vi "H-cube - MAIN.vi"() -> ()   [LabVIEW 2019]
doc: "Use this template to build a producer/consumer design pattern with events to produce queue items. Use this design pattern instead of the User Interface Event Handler pattern for user interfaces when you want to execute code asynchronously in response to an event without slowing the user interface responsiveness."
uses:
  MAIN STATUS.ctl
  FPGA/FPGA.ctl
  FPGA/ResultSweep.vi
  <vilib>/Utility/file.llb/Write Delimited Spreadsheet (DBL).vi
  FPGA/FPGA.lvlib
panel:
  in  "ClearFIFO":bool
  in  "FIFO EN":bool
  out "FIFO":string[][](array[string])
  in  "Add FIFO":bool
  in  "Continuous save":bool
  in  "File name":string
  in  "Path":path
  in  "Incremental Save":bool
  in  "Continuous run":bool
  in  "raw data slice":bool
  in  "Settling at step time":enum16{"99%", "99,9%"}(ring)=enum."99,9%"
  in  "Lockin filter order":u32=2 min=1 max=4
  out "Averaging":bool
  in  "Averaging":bool
  out "Averaging prefered":bool
  in  "Auto MA selection":bool
  out "Number of steps":i32=1
  in  "Save":bool caption="OK Button"
  in  "Digital Gain":i32(ring) items=["1", "2", "4", "8", "16", "32", "64"]
  out "XY Graph 2":cluster{dbl[], dbl[]}(graph)
  out "XY Graph":cluster{dbl[], dbl[]}(graph)
  in  "DAC-ADC Latency":u16=80 min=1 max=1024 step=1
  out "Acquiring":bool
  in  "Lock-in":bool=TRUE
  in  "Amplitude [mVpp]":dbl=100.0 min=0.0 max=5000.0
  in  "connect":bool
  out "Connected":bool=TRUE
  out "Sweep speed [Hz/s]":dbl=999.9995081132196
  out "Time for step [ms]":dbl=100.0
  in  "Discrete\nsweep":bool=TRUE
  in  "Freq. step [Hz]":dbl=100.0 min=0.0
  in  "Sweep duration [s]":dbl=10.0 min=0.0
  in  "Stop freq. [Hz]":dbl=20000.0
  in  "Start freq. [Hz]":dbl=10000.0
  in  "exit":bool
  in  "stop":bool
  in  "start":bool
  # "SWEEP\nCONTROLS"
  # "ADVANCED\nCONTROLS"
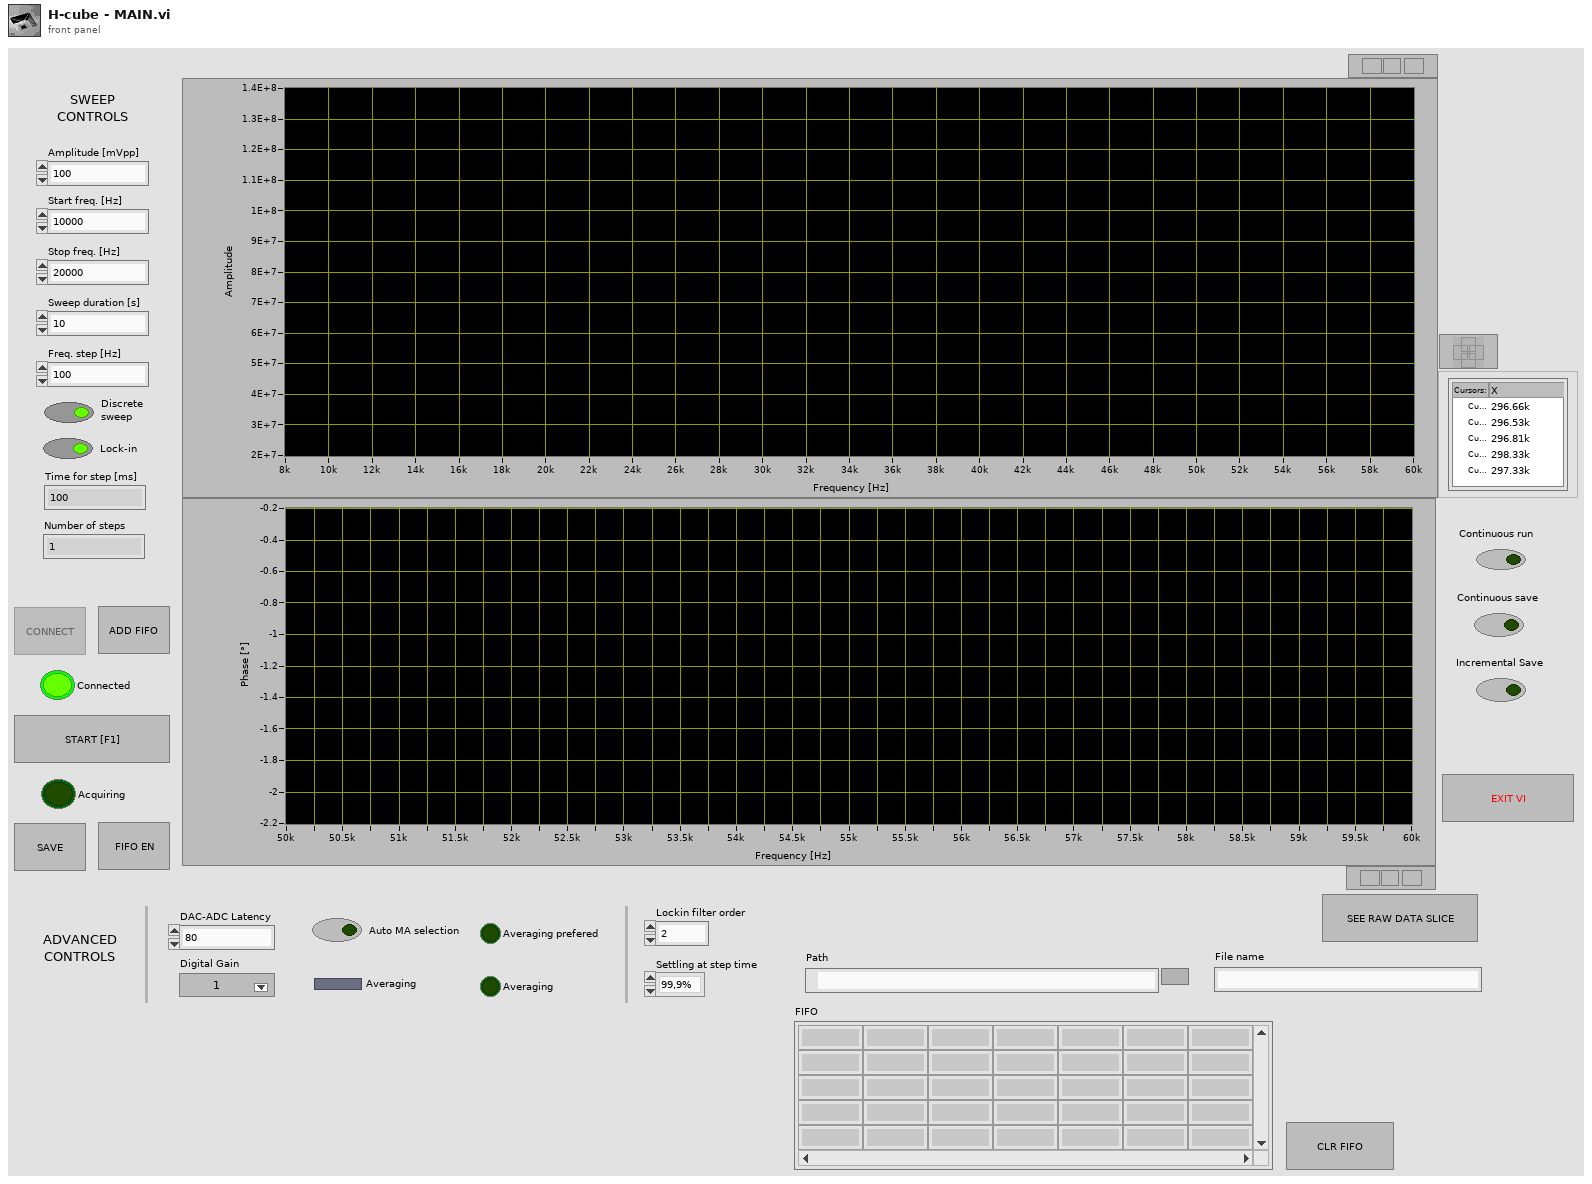
[diagram p1: front panel]
types:
  T1 = enum8{"Enabled", "Disabled", "Disabled and Grayed Out"}
  T2 = typedef "MAIN STATUS.ctl" = enum16{"IDLE", "Refresh UI", "ChangeParameters", "StopSweep", "StartSweep", "RawData", "CheckParameters", "SendParameters", "Connect", "AddFIFO", "Save", "Quit", "ClrFIFO", "StartSweepFIFO"}
  T3 = typedef "FPGA.lvlib/FPGA.ctl" = cluster{"Start freq. [Hz]":dbl, "Sweep duration [s]":dbl, "Freq. step [Hz]":dbl, "DAC Sample Rate":dbl, "ADC Sample Rate":dbl, "CMD port":u16, "DFAST port":u16, "CMD ID":refnum<k16>, "DFAST ID":refnum<k16>, "CMD error out":errorcluster, "FPGA IP":string, "DFAST error out ":errorcluster, "Stop freq. [Hz]":dbl, "Discrete sweep":bool, "Initial NCO":u32, "Difference NCO":i32, "step NCO":i64, "Final NCO":u32, "clocks for step":u32, "demodulation":bool, "NCO Phase Precision":u32, "NCO Sample Rate":dbl, "Time for step [s]":dbl, "NCO freq. resolution":dbl, "Sweep speed [Hz/s]":dbl, "Connected":bool, "Slew Rate [V/us]":dbl, "Parameters_ok":bool, "Amplitude [mVpp]":dbl, "Scale Factor":fxp<+,16,0>, "Acquiring":bool, "DAC-ADC Latency":u16, "Digital Gain":i32, "Number of steps":i32, "Averaging preferred":bool, "Filter Order":u32, "Settling":enum16{"99%", "99,9%"}, "FIFO":cluster{"Start freq. [Hz]":dbl, "Sweep duration [s]":dbl, "Freq. step [Hz]":dbl, "Stop freq. [Hz]":dbl, "Time for step [s]":dbl, "Amplitude [mVpp]":dbl, "Number of steps":i32}[]}
  T4 = cluster{"CMD port":u16, "CMD ID":refnum<k16>, "DFAST port":u16, "DFAST ID":refnum<k16>, "CMD error out":errorcluster, "DFAST error out ":errorcluster, "FPGA IP":string}
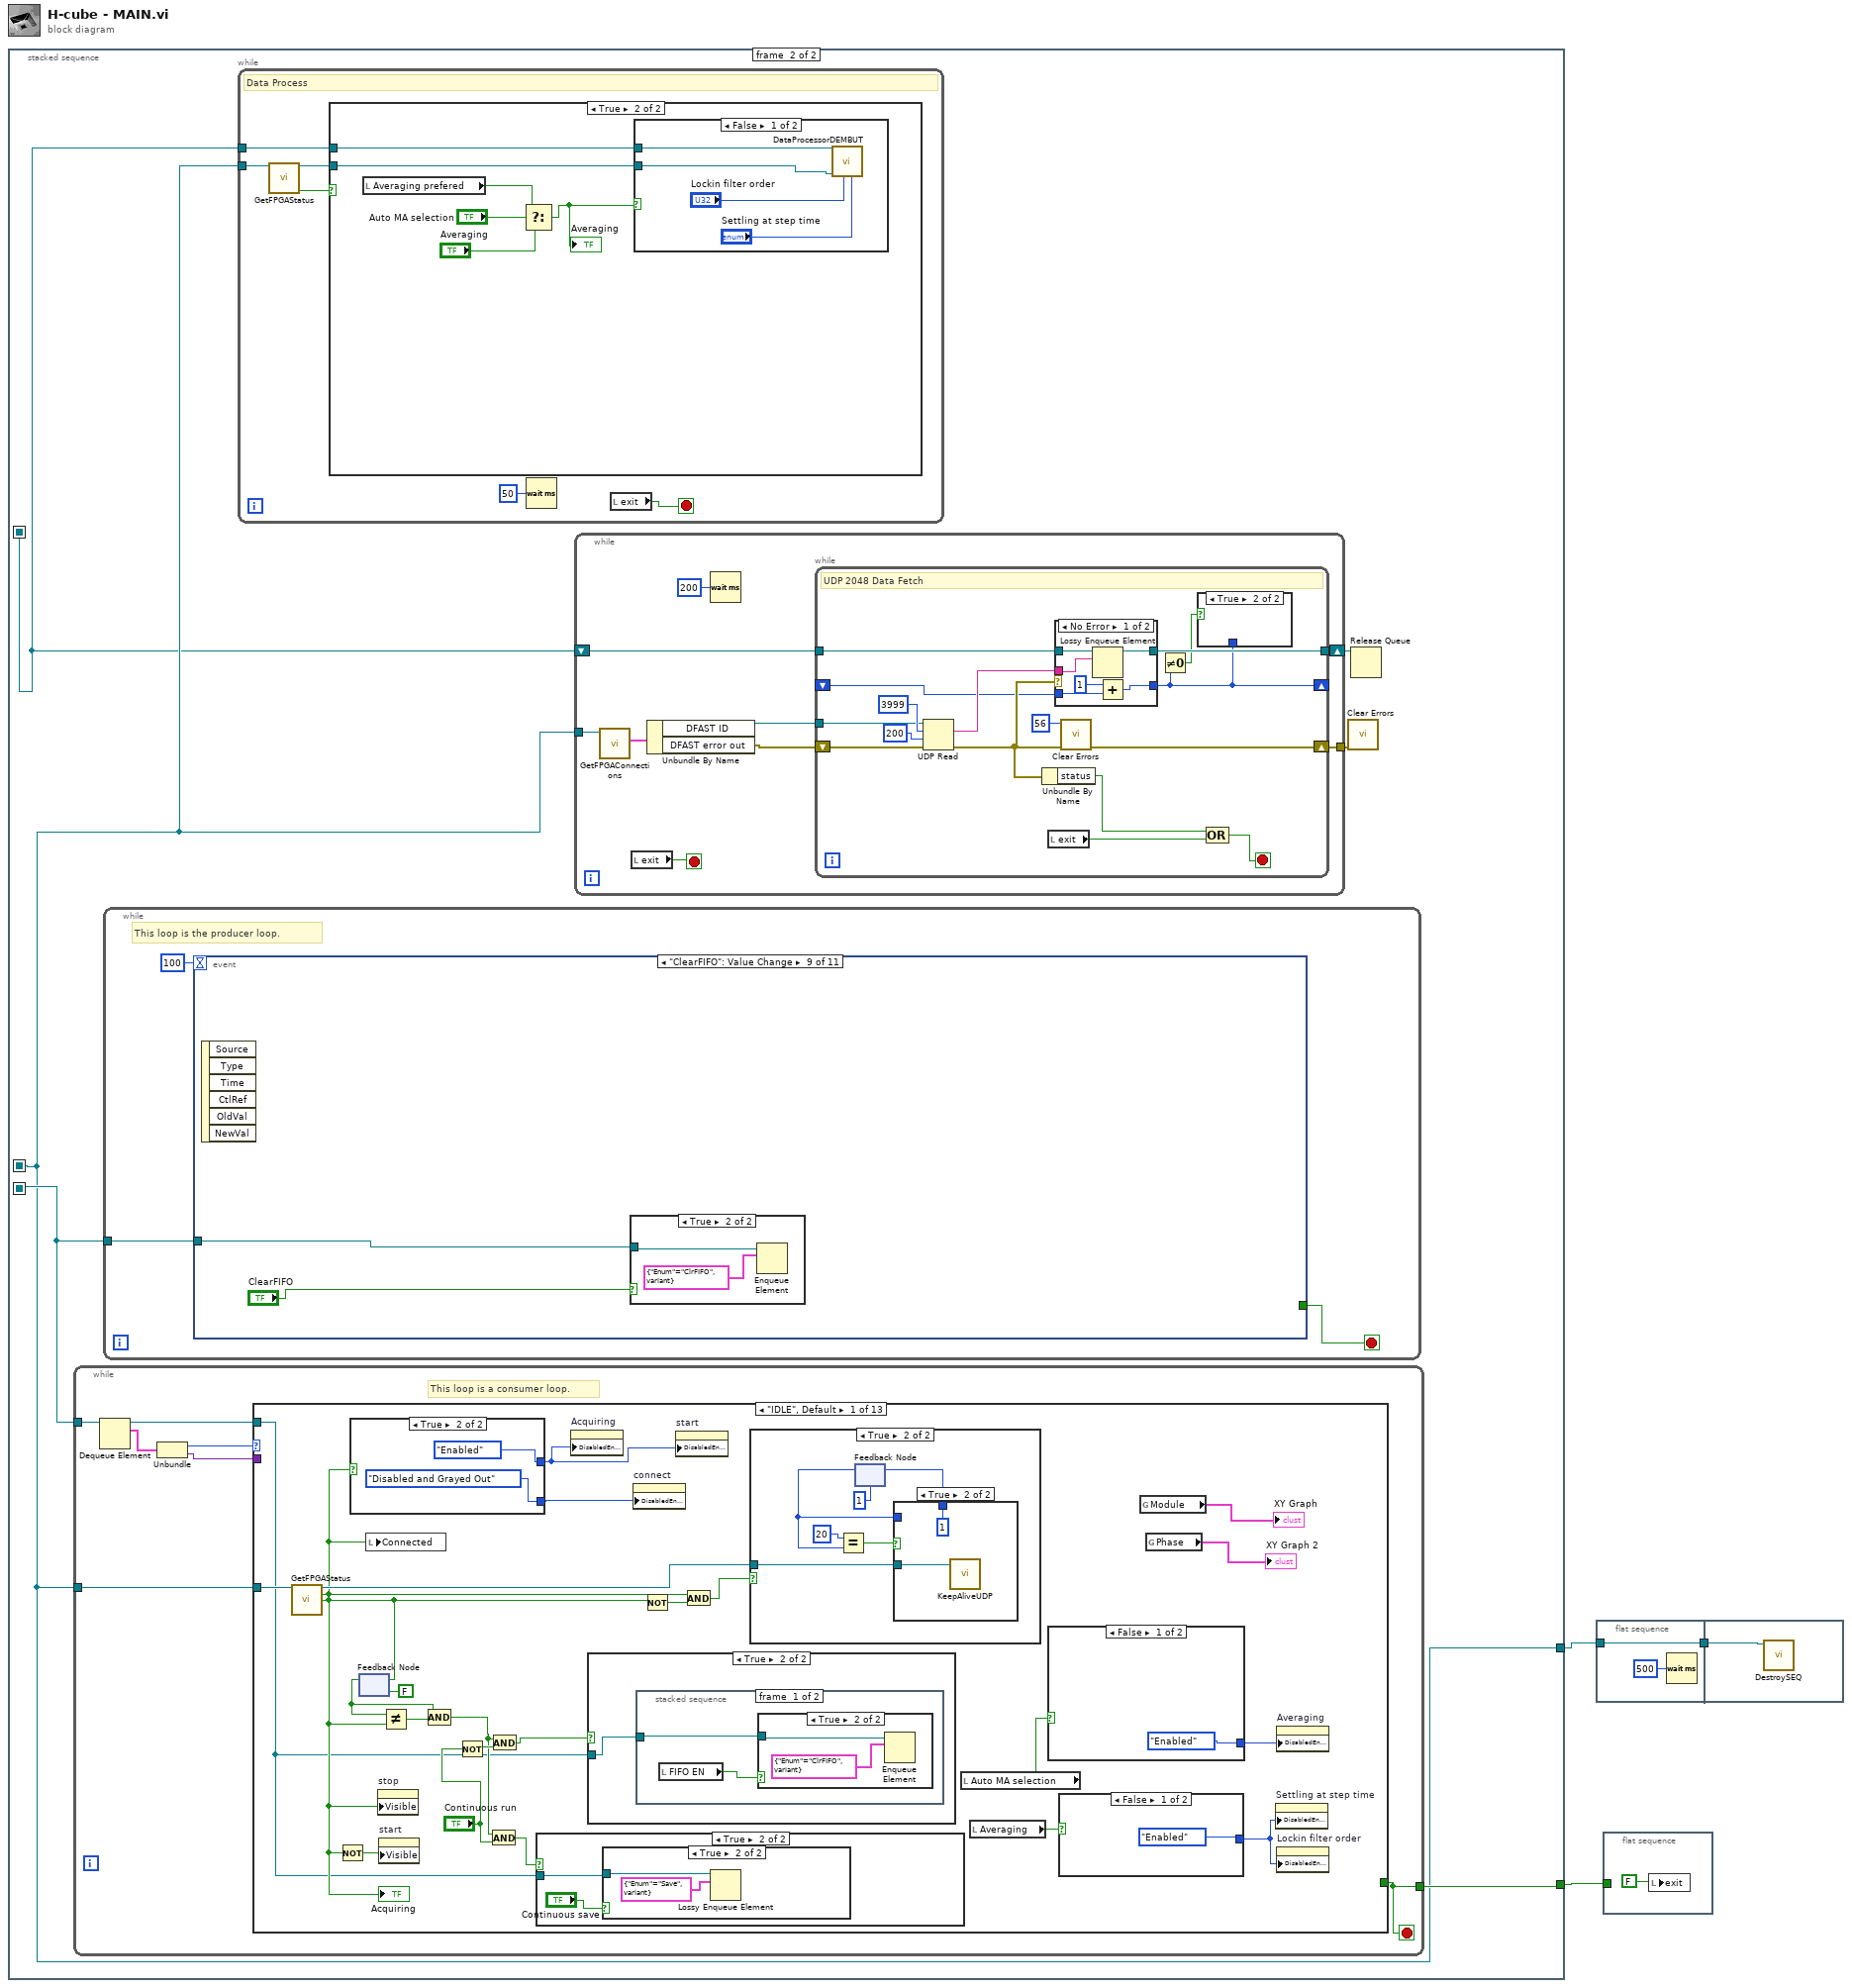
[diagram p0: block diagram]
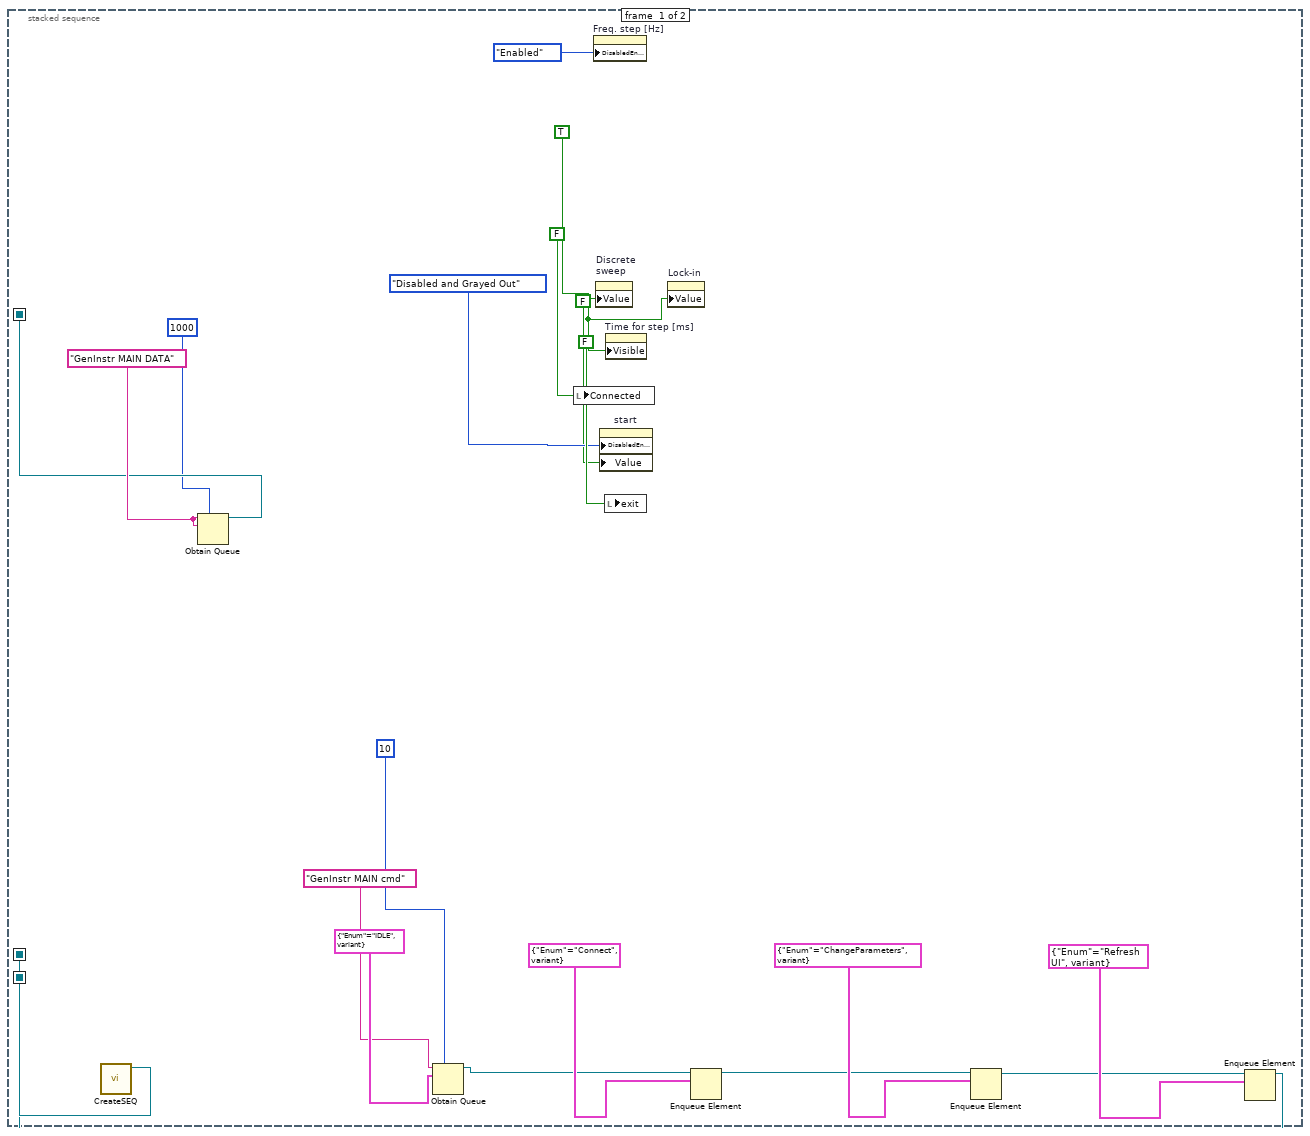
[diagram p2: hidden frame]
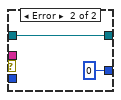
[diagram p4: hidden frame]
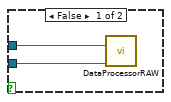
[diagram p5: hidden frame]
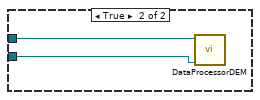
[diagram p6: hidden frame]
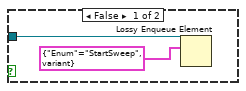
[diagram p8: hidden frame]
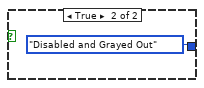
[diagram p9: hidden frame]
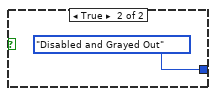
[diagram p10: hidden frame]
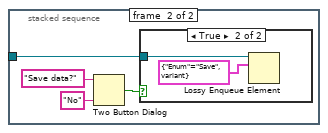
[diagram p13: hidden frame]
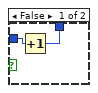
[diagram p16: hidden frame]
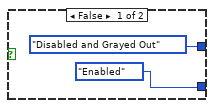
[diagram p17: hidden frame]
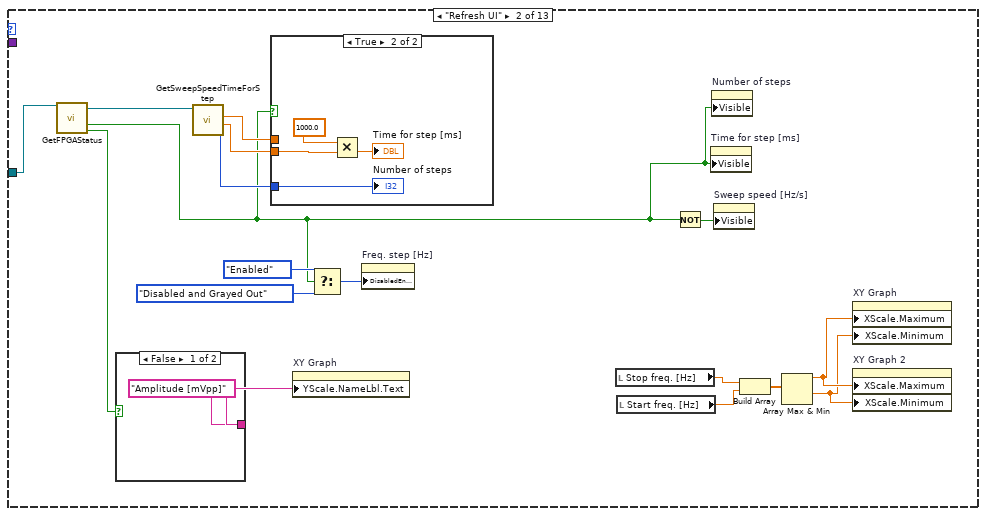
[diagram p18: hidden frame]
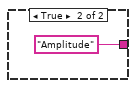
[diagram p19: hidden frame]
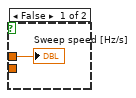
[diagram p20: hidden frame]
diagram:
  n1 = stacked-sequence {
    seq-local: [w11 _] -> [_ w29]
    seq-local: [w19 _] -> [_ w24]
    seq-local: [w15 _] -> [_ w25]
    tunnel: [_ w28] -> w3
    tunnel: [_ w25] -> w2
    frame #0 {
      w4 = TRUE ("Discrete\nsweep")
      w20 = "GenInstr MAIN DATA" ("name (unnamed)")
      n2 = call "CreateSEQ.vi"() -> ("FPGA out"=w15:refnum<queue>)  [unwired: 10 in, 1 out]
      n3 = Obtain Queue(max queue size (-1, unlimited)=1000, name (unnamed)=w20, element data type=w20) -> (queue out=w19:refnum<queue>)  [unwired: 2 in, 2 out]
      n4 = Obtain Queue(max queue size (-1, unlimited)=10, name (unnamed)="GenInstr MAIN cmd", element data type=cluster{"Enum":T2, variant} {"Enum"=enum."IDLE", variant}) -> (queue out=w9:refnum<queue>)  [unwired: 2 in, 2 out]
      n5 = local write "Connected"(FALSE ("Connected")) -> ()
      n6 = property on="Freq. step [Hz]" class="DigNum (strict)"("DisabledEnum"=T1."Enabled" ("Disabled")) -> ()  [unwired: 2 in, 2 out]
      n7 = property on="Discrete\nsweep" class="Bool (strict)"("Value"=w4) -> ()  [unwired: 2 in, 2 out]
      n8 = property on="start" class="Bool"("DisabledEnum"=T1."Disabled and Grayed Out" ("Disabled"), "Value"=FALSE ("start")) -> ()  [unwired: 2 in, 2 out]
      n9 = local write "exit"(FALSE ("stop")) -> ()
      n10 = property on="Time for step [ms]" class="DigNum (strict)"("Visible"=w4) -> ()  [unwired: 2 in, 2 out]
      n11 = property on="Lock-in" class="Bool (strict)"("Value"=w4) -> ()  [unwired: 2 in, 2 out]
      n12 = Enqueue Element(queue=w9, element=cluster{"Enum":T2, variant} {"Enum"=enum."Connect", variant}) -> (queue out=w8:refnum<queue>)  [unwired: 2 in, 2 out]
      n13 = Enqueue Element(queue=w8, element=cluster{"Enum":T2, variant} {"Enum"=enum."ChangeParameters", variant}) -> (queue out=w12:refnum<queue>)  [unwired: 2 in, 2 out]
      n14 = Enqueue Element(queue=w12, element=cluster{"Enum":T2, variant} {"Enum"=enum."Refresh UI", variant}) -> (queue out=w11:refnum<queue>)  [unwired: 2 in, 2 out]
    }
    frame #1 {
      n15 = while {
        tunnel: w29 -> [w84]
        tunnel: [w86] -> w28
        tunnel: w25 -> [w85]
        stop <- w86 stop-if-true
        # "This loop is a consumer loop."
        n16 = Dequeue Element(queue=w84) -> (queue out=w83:refnum<queue>, element=w89:cluster{"Enum":T2, variant})  [unwired: 2 in, 2 out]
        n17 = Unbundle(w89) -> ("Enum"=w88:T2, w87:variant)
        n18 = case shown="\"IDLE\", Default" w88 {
          tunnel: [_ _ TRUE _ _ _ _ _ _ _ _ _ _] -> w86
          tunnel: w87 -> [_ _ _ _ _ _ _ _ _ _ _ _ _]
          tunnel: w85 -> [w113 w158 w175 _ w219 w232 w239 _ w246 _ w253 w256 w258]
          tunnel: w83 -> [w90 _ _ w183 _ w230 _ _ _ _ _ _ _]
          frame "IDLE", Default {
            n19 = call "GetFPGAStatus.vi"("FPGA in"=w113) -> ("FPGA out"=w110:refnum<queue>, "Connected"=w97:bool, "Acquiring"=w105:bool)  [unwired: 9 in, 3 out]
            "Acquiring" <- w105
            n20 = Not(x=w105) -> (.not. x?=w107:bool)
            n21 = case shown="True" w97 {
              tunnel: [T1."Disabled and Grayed Out" ("Disabled") T1."Enabled" ("Disabled")] -> w98
              tunnel: [T1."Enabled" ("Disabled") T1."Disabled and Grayed Out" ("Disabled")] -> w96
              frame False {
              }
              frame True {
              }
            }
            n22 = feedback-in #1(w105) -> ()
            n23 = feedback #1(FALSE ("Acquiring")) -> (w104:bool)
            n24 = local write "Connected"(w97) -> ()
            n25 = property on="stop" class="Bool"("Visible"=w105) -> ()  [unwired: 2 in, 2 out]
            n26 = property on="start" class="Bool"("Visible"=w107) -> ()  [unwired: 2 in, 2 out]
            n27 = Not Equal?(x=w104, y=w105) -> (x != y?=w103:bool)
            n28 = Compound Arithmetic op=AND(w104, w103) -> (w92:bool)
            n29 = Not(x="Continuous run") -> (.not. x?=w94:bool)
            n30 = And(x=w92, y="Continuous run") -> (x .and. y?=w91:bool)
            n31 = And(x=w92, y=w94) -> (x .and. y?=w95:bool)
            n32 = case shown="True" w91 {
              tunnel: w90 -> [_ w114]
              frame False {
              }
              frame True {
                n33 = case shown="True" "Continuous save" {
                  tunnel: w114 -> [w116 w118]
                  frame False {
                    n34 = Lossy Enqueue Element(queue=w116, element=cluster{"Enum":T2, variant} {"Enum"=enum."StartSweep", variant}) -> ()  [unwired: 1 in, 4 out]
                  }
                  frame True {
                    n35 = Lossy Enqueue Element(queue=w118, element=cluster{"Enum":T2, variant} {"Enum"=enum."Save", variant}) -> ()  [unwired: 1 in, 4 out]
                  }
                }
              }
            }
            n36 = property on="Acquiring" class="Bool (strict)"("DisabledEnum"=w98) -> ()  [unwired: 2 in, 2 out]
            n37 = case shown="True" w95 {
              tunnel: w90 -> [_ w124]
              frame False {
              }
              frame True {
                n38 = stacked-sequence {
                  tunnel: w124 -> [w126 w129]
                  frame #0 {
                    n39 = local read "FIFO EN"() -> (w125:bool)
                    n40 = case shown="True" w125 {
                      tunnel: w126 -> [_ w127]
                      frame False {
                      }
                      frame True {
                        n41 = Enqueue Element(queue=w127, element=cluster{"Enum":T2, variant} {"Enum"=enum."ClrFIFO", variant}) -> ()  [unwired: 2 in, 3 out]
                      }
                    }
                  }
                  frame #1 {
                    n42 = Two Button Dialog(message="Save data?", 1:"No" ("F button name (\"Cancel\")")) -> (T button?=w130:bool)  [unwired: 1 in]
                    n43 = case shown="True" w130 {
                      tunnel: w129 -> [_ w133]
                      frame False {
                      }
                      frame True {
                        n44 = Lossy Enqueue Element(queue=w133, element=cluster{"Enum":T2, variant} {"Enum"=enum."Save", variant}) -> ()  [unwired: 1 in, 4 out]
                      }
                    }
                  }
                }
              }
            }
            n45 = property on="connect" class="Bool"("DisabledEnum"=w96) -> ()  [unwired: 2 in, 2 out]
            n46 = Not(x=w105) -> (.not. x?=w111:bool)
            n47 = property on="start" class="Bool"("DisabledEnum"=w98) -> ()  [unwired: 2 in, 2 out]
            n48 = And(x=w97, y=w111) -> (x .and. y?=w112:bool)
            n49 = case shown="True" w112 {
              tunnel: w110 -> [_ w136]
              frame False {
              }
              frame True {
                n50 = feedback #2(1 ("y")) -> (w135:i32)
                n51 = Equal?(x=20 ("y"), y=w135) -> (x = y?=w138:bool)
                n52 = case shown="True" w138 {
                  tunnel: [w141 1] -> w137
                  tunnel: w135 -> [w142 _]
                  tunnel: w136 -> [_ w144]
                  frame False {
                    n53 = Increment(x=w142) -> (x+1=w141:i32)
                  }
                  frame True {
                    n54 = call "KeepAliveUDP.vi"("FPGA in"=w144) -> ()  [unwired: 10 in, 1 out]
                  }
                }
                n55 = feedback-in #2(w137) -> ()
              }
            }
            n56 = local read "Auto MA selection"() -> (w100:bool)
            n57 = local read "Averaging"() -> (w102:bool)
            n58 = case shown="False" w100 {
              tunnel: [T1."Enabled" ("Disabled") T1."Disabled and Grayed Out" ("Disabled")] -> w101
              frame False {
              }
              frame True {
              }
            }
            n59 = case shown="False" w102 {
              tunnel: [T1."Enabled" ("Disabled") T1."Disabled and Grayed Out" ("Disabled")] -> w99
              frame False {
              }
              frame True {
              }
            }
            n60 = global read "ResultSweep.vi" "Module"() -> (→"XY Graph":cluster{dbl[], dbl[]})
            n61 = global read "ResultSweep.vi" "Phase"() -> (→"XY Graph 2":cluster{dbl[], dbl[]})
            n62 = property on="Settling at step time" class="Enum (strict)"("DisabledEnum"=w99) -> ()  [unwired: 2 in, 2 out]
            n63 = property on="Averaging" class="Bool (strict)"("DisabledEnum"=w101) -> ()  [unwired: 2 in, 2 out]
            n64 = property on="Lockin filter order" class="DigNum (strict)"("DisabledEnum"=w99) -> ()  [unwired: 2 in, 2 out]
          }
          frame "Refresh UI" {
            n65 = call "GetFPGAStatus.vi"("FPGA in"=w158) -> ("FPGA out"=w157:refnum<queue>, "Discrete Sweep"=w149:bool, "Demodulation"=w156:bool)  [unwired: 9 in, 3 out]
            n66 = case shown="False" w156 {
              tunnel: ["Amplitude [mVpp]" ("X Scale.Name Label.Text") "Amplitude" ("X Scale.Name Label.Text")] -> w159
              frame False {
              }
              frame True {
              }
            }
            n67 = call "GetSweepSpeedTimeForStep.vi"("FPGA in"=w157) -> ("Number of steps"=w150:i32, "Time for step [s]"=w162:dbl, "Sweep speed [Hz/s]"=w160:dbl)  [unwired: 7 in, 1 out]
            n68 = case shown="True" w149 {
              tunnel: w162 -> [_ w172]
              tunnel: w160 -> [w168 _]
              tunnel: w150 -> [_ w169]
              frame False {
                "Sweep speed [Hz/s]" <- w168
              }
              frame True {
                n69 = Multiply(x=1000.0, y=w172) -> (x*y=→"Time for step [ms]":dbl)
                "Number of steps" <- w169
              }
            }
            n70 = property on="XY Graph" class="XYGraph (strict)"("YScale.NameLbl.Text"=w159) -> ()  [unwired: 2 in, 2 out]
            n71 = Select(t=T1."Enabled", s=w149, f=T1."Disabled and Grayed Out" ("Disabled")) -> (s? t:f=w165:T1)
            n72 = property on="Freq. step [Hz]" class="DigNum (strict)"("DisabledEnum"=w165) -> ()  [unwired: 2 in, 2 out]
            n73 = local read "Stop freq. [Hz]"() -> (w154:dbl)
            n74 = local read "Start freq. [Hz]"() -> (w153:dbl)
            n75 = Not(x=w149) -> (.not. x?=w161:bool)
            n76 = property on="Time for step [ms]" class="DigNum (strict)"("Visible"=w149) -> ()  [unwired: 2 in, 2 out]
            n77 = property on="Number of steps" class="DigNum (strict)"("Visible"=w149) -> ()  [unwired: 2 in, 2 out]
            n78 = property on="Sweep speed [Hz/s]" class="DigNum (strict)"("Visible"=w161) -> ()  [unwired: 2 in, 2 out]
            n79 = Build Array(w154, w153) -> (w155:dbl[])
            n80 = Array Max & Min(array=w155) -> (max value=w152:dbl, min value=w151:dbl)  [unwired: 2 out]
            n81 = property on="XY Graph" class="XYGraph (strict)"("XScale.Maximum"=w152, "XScale.Minimum"=w151) -> ()  [unwired: 2 in, 2 out]
            n82 = property on="XY Graph 2" class="XYGraph (strict)"("XScale.Maximum"=w152, "XScale.Minimum"=w151) -> ()  [unwired: 2 in, 2 out]
          }
          frame "Quit" {
            n83 = call "GetFPGAStatus.vi"("FPGA in"=w175) -> ("FPGA out"=w174:refnum<queue>, "Acquiring"=w173:bool)  [unwired: 9 in, 4 out]
            n84 = case shown="False" w173 {
              tunnel: [w178 w180] -> w176
              tunnel: w174 -> [w178 w179]
              frame False {
              }
              frame True {
                n85 = call "StopSweep.vi"("FPGA in"=w179) -> ("FPGA out"=w180:refnum<queue>)  [unwired: 10 in]
              }
            }
            n86 = call "DisconnectUDP.vi"("FPGA in"=w176) -> ()  [unwired: 10 in, 1 out]
          }
          frame "Save" {
            n87 = local read "Continuous save"() -> (w181:bool)
            n88 = Or(x="Incremental Save", y=w181) -> (x .or. y?=w182:bool)
            n89 = case shown="False" w182 {
              tunnel: [w196 w204] -> w186
              tunnel: w183 -> [_ w199]
              frame False {
                n90 = call "File Dialog"("pattern (all files)"="*.hcube" ("pattern label"), "pattern label"="hcube") -> ("selected path"=w196:path)  [unwired: 10 in, 3 out]
              }
              frame True {
                n91 = Concatenate Strings("File name", ".hcube" ("string")) -> (w202:string)
                n92 = Build Path(base path="Path", name or relative path=w202) -> (appended path=w205:path)
                n93 = call <vilib>:"Create File with Incrementing Suffix.vi"("format string (\" (%d)\")"="_%04d" ("format string (\" (%d)\")"), "file path"=w205) -> ("actual path"=w204:path, "refnum out"=w197:refnum<file>)  [unwired: 7 in, 1 out]
                n94 = Enqueue Element(queue=w199, element=cluster{"Enum":T2, variant} {"Enum"=enum."StartSweep", variant}) -> ()  [unwired: 2 in, 3 out]
                n95 = Close File(refnum=w197) -> ()  [unwired: 1 in, 2 out]
              }
            }
            n96 = global read "ResultSweep.vi" "Module"() -> (w193:cluster{dbl[], dbl[]})
            n97 = global read "ResultSweep.vi" "Phase"() -> (w192:cluster{dbl[], dbl[]})
            n98 = Unbundle(w192) -> (w189:dbl[])  [unwired: 1 out]
            n99 = Unbundle(w193) -> (w191:dbl[], w190:dbl[])
            n100 = Build Array(w191, w190, w189) -> (w188:dbl[][])
            n101 = call-poly <vilib>:"Write Delimited Spreadsheet.vi"("file path (dialog if empty)"=w186, "format (%.3f)"="%e", "2D data"=w188, "transpose? (no:F)"=TRUE) -> ()  [unwired: 10 in, 2 out]
          }
          frame "ChangeParameters" {
            n102 = local read "DAC-ADC Latency"() -> (w213:u16)
            n103 = local read "Sweep duration [s]"() -> (w223:dbl)
            n104 = local read "Stop freq. [Hz]"() -> (w222:dbl)
            n105 = local read "Discrete\nsweep"() -> (w225:bool)
            n106 = local read "Freq. step [Hz]"() -> (w224:dbl)
            n107 = local read "Start freq. [Hz]"() -> (w221:dbl)
            n108 = local read "Amplitude [mVpp]"() -> (w220:dbl)
            n109 = local read "Lock-in"() -> (w214:bool)
            n110 = local read "Digital Gain"() -> (w212:i32)
            n111 = Bundle By Name(cluster=T3 {"Start freq. [Hz]"=10.0, "Sweep duration [s]"=0.1, "Freq. step [Hz]"=0.1, "DAC Sample Rate"=1388888.8888, "ADC Sample Rate"=50000000.0, "CMD port"=2047, "DFAST port"=2048, "CMD ID"=refnum, "DFAST ID"=refnum, "CMD error out"={"status"=FALSE, "code"=0, "source"=""}, "FPGA IP"="192.168.1.12", "DFAST error out "={"status"=FALSE, "code"=0, "source"=""}, "Stop freq. [Hz]"=0.0, "Discrete sweep"=FALSE, "Initial NCO"=10, "Difference NCO"=0, "step NCO"=0, "Final NCO"=0, "clocks for step"=0, "demodulation"=FALSE, "NCO Phase Precision"=32, "NCO Sample Rate"=50000000.0, "Time for step [s]"=0.1, "NCO freq. resolution"=32.0, "Sweep speed [Hz/s]"=0.1, "Connected"=FALSE, "Slew Rate [V/us]"=50000000.0, "Parameters_ok"=FALSE, "Amplitude [mVpp]"=10.0, "Scale Factor"=0.999969482421875, "Acquiring"=FALSE, "DAC-ADC Latency"=1, "Digital Gain"=0, "Number of steps"=1, "Averaging preferred"=FALSE, "Filter Order"=1, "Settling"=enum."99,9%", "FIFO"=[]} ("FPGA CLUSTER"), "Start freq. [Hz]"=w221, "Stop freq. [Hz]"=w222, "Sweep duration [s]"=w223, "Freq. step [Hz]"=w224, "Discrete sweep"=w225, "Amplitude [mVpp]"=w220, "demodulation"=w214, "DAC-ADC Latency"=w213, "Digital Gain"=w212) -> (w218:T3)
            n112 = call "CheckParams.vi"("FPGA CLUSTER"=w218, "FPGA in"=w219) -> ("FPGA out"=w211:refnum<queue>)  [unwired: 8 in, 1 out]
            n113 = call "GetFPGAStatus.vi"("FPGA in"=w211) -> ("FPGA out"=w210:refnum<queue>, "Connected"=w209:bool, "Parameters Ok"=w208:bool)  [unwired: 9 in, 3 out]
            n114 = And(x=w209, y=w208) -> (x .and. y?=w207:bool)
            n115 = case shown="True" w207 {
              tunnel: w210 -> [_ w229]
              frame False {
              }
              frame True {
                n116 = call "UpdateParams.vi"("FPGA in"=w229) -> ("FPGA out"=w228:refnum<queue>)  [unwired: 10 in]
                n117 = call "CheckAveragingDEM.vi"("FPGA in"=w228) -> ("Averaging"=→"Averaging prefered":bool)  [unwired: 7 in, 1 out]
              }
            }
            n118 = Select(t=T1."Enabled" ("Disabled"), s=w207, f=T1."Disabled and Grayed Out" ("Disabled")) -> (s? t:f=w217:T1)
            n119 = property on="start" class="Bool"("DisabledEnum"=w217) -> ()  [unwired: 2 in, 2 out]
          }
          frame "Connect" {
            n120 = call "ConnectUDP.vi"("FPGA in"=w232) -> ("Connected"=w231:bool)  [unwired: 9 in, 1 out]
            "Connected" <- w231
            n121 = case shown="True" w231 {
              tunnel: w230 -> [_ w233]
              frame False {
              }
              frame True {
                n122 = Enqueue Element(queue=w233, element=cluster{"Enum":T2, variant} {"Enum"=enum."ChangeParameters", variant}) -> (queue out=w236:refnum<queue>)  [unwired: 2 in, 2 out]
                n123 = Enqueue Element(queue=w236, element=cluster{"Enum":T2, variant} {"Enum"=enum."Refresh UI", variant}) -> ()  [unwired: 2 in, 3 out]
              }
            }
          }
          frame "StartSweep" {
            n124 = flat-sequence {
              tunnel: w239 -> [w241]
              tunnel: [w240] -> w238
              tunnel: w238 -> [w243]
              tunnel: [w243] -> w237
              tunnel: w237 -> [w245]
              frame #0 {
                n125 = call "SendParameters.vi"("FPGA in"=w241) -> ("FPGA out"=w240:refnum<queue>)  [unwired: 10 in]
              }
              frame #1 {
                n126 = Wait (ms)(milliseconds to wait=u32 20) -> ()  [unwired: 1 out]
              }
              frame #2 {
                n127 = call "StartSweep.vi"("FIFO enabled"="FIFO EN", "FPGA in"=w245) -> ()  [unwired: 9 in, 1 out]
              }
            }
          }
          frame "CheckParameters" {
          }
          frame "StopSweep" {
            n128 = call "StopSweep.vi"("FPGA in"=w246) -> ()  [unwired: 10 in, 1 out]
          }
          frame "RawData" {
            n129 = local read "Lock-in"() -> (w247:bool)
            n130 = case shown="True" w247 {
              tunnel: ["FPGA.lvlib:DataProcessorRAW.vi" "FPGA.lvlib:DataProcessorDEMBUT.vi"] -> w249
              frame False {
              }
              frame True {
              }
            }
            n131 = Open VI Reference(vi path=w249) -> (vi reference=w250:refnum<vi>)  [unwired: 5 in, 1 out]
            n132 = invoke class="VI" method="FP.Open"(reference=w250) -> (reference out=w248:refnum<vi>)  [unwired: 4 in, 4 out]
            n133 = Close Reference(reference=w248) -> ()  [unwired: 1 in, 1 out]
          }
          frame "SendParameters" {
            n134 = call "SendParameters.vi"("FPGA in"=w253) -> ()  [unwired: 10 in, 1 out]
          }
          frame "AddFIFO" {
            n135 = call "SendParameters.vi"("FPGA in"=w256) -> ("FPGA out"=w255:refnum<queue>)  [unwired: 10 in]
            n136 = call "AddFIFO.vi"("FPGA in"=w255) -> ("Table"=→"FIFO":string[][])  [unwired: 9 in, 1 out]
          }
          frame "ClrFIFO" {
            n137 = call "ClrFIFO.vi"("FPGA in"=w258) -> ("Table"=w257:string[][])  [unwired: 9 in, 1 out]
            n138 = local write "FIFO"(w257) -> ()
          }
        }
      }
      n139 = while {
        tunnel: w29 -> [w261]
        stop <- w259 stop-if-true
        # "This loop is the producer loop."
        n140 = event shown="[8] \"ClearFIFO\": Value Change" {
          selector: _ -> [_ _ _ _ _ _ _ _ _ _ _]
          dyn-events: _ -> [_ _ _ _ _ _ _ _ _ _ _]
          timeout: 100 -> [_ _ _ _ _ _ _ _ _ _ _]
          tunnel: w261 -> [w266 w269 w272 w275 w280 w284 w288 w290 w294 w299 _]
          tunnel: [_ _ _ _ _ "exit" _ _ _ _ _] -> w259
          event Timeout {
            n141 = event-data() -> ()  [unwired: 1 in, 1 out]
            n142 = Get Queue Status(queue=w266) -> (queue out=w265:refnum<queue>, # pending remove=w264:i32)  [unwired: 2 in, 6 out]
            n143 = Less?(x=w264, y=3) -> (x < y?=w262:bool)
            n144 = case shown="True" w262 {
              tunnel: w265 -> [_ w268]
              frame False {
              }
              frame True {
                n145 = Enqueue Element(queue=w268, element=cluster{"Enum":T2, variant} {"Enum"=enum."IDLE", variant}) -> ()  [unwired: 2 in, 3 out]
              }
            }
          }
          event "connect": Value Change {
            n146 = event-data() -> ()  [unwired: 1 in, 1 out]
            n147 = Enqueue Element(queue=w269, element=cluster{"Enum":T2, variant} {"Enum"=enum."Connect", variant}) -> ()  [unwired: 2 in, 3 out]
          }
          event "start": Value Change {
            n148 = event-data() -> ()  [unwired: 1 in, 1 out]
            n149 = case shown="True" "start" {
              tunnel: w272 -> [_ w274]
              frame False {
              }
              frame True {
                n150 = Enqueue Element(queue=w274, element=cluster{"Enum":T2, variant} {"Enum"=enum."StartSweep", variant}) -> ()  [unwired: 2 in, 3 out]
              }
            }
          }
          event "raw data slice": Value Change {
            n151 = event-data() -> ()  [unwired: 1 in, 1 out]
            n152 = case shown="True" "raw data slice" {
              tunnel: w275 -> [_ w278]
              frame False {
              }
              frame True {
                n153 = Enqueue Element(queue=w278, element=cluster{"Enum":T2, variant} {"Enum"=enum."RawData", variant}) -> ()  [unwired: 2 in, 3 out]
              }
            }
          }
          event "stop": Value Change {
            n154 = event-data() -> ()  [unwired: 1 in, 1 out]
            n155 = case shown="False" "stop" {
              tunnel: w280 -> [_ w282]
              frame False {
              }
              frame True {
                n156 = Enqueue Element(queue=w282, element=cluster{"Enum":T2, variant} {"Enum"=enum."StopSweep", variant}) -> ()  [unwired: 2 in, 3 out]
              }
            }
          }
          event "exit": Value Change {
            n157 = event-data() -> ()  [unwired: 1 in, 1 out]
            n158 = Enqueue Element(queue=w284, element=cluster{"Enum":T2, variant} {"Enum"=enum."Quit", variant}) -> ()  [unwired: 2 in, 3 out]
          }
          event "Start freq. [Hz]", "Stop freq. [Hz]", "Sweep duration [s]", "Freq. step [Hz]", "Discrete\nsweep", "Amplitude [mVpp]", "Lock-in", "DAC-ADC Latency", "Digital Gain": Value Change {
            n159 = event-data() -> ()  [unwired: 1 in, 6 out]
            n160 = Enqueue Element(queue=w288, element=cluster{"Enum":T2, variant} {"Enum"=enum."ChangeParameters", variant}) -> (queue out=w286:refnum<queue>)  [unwired: 2 in, 2 out]
            n161 = Enqueue Element(queue=w286, element=cluster{"Enum":T2, variant} {"Enum"=enum."Refresh UI", variant}) -> ()  [unwired: 2 in, 3 out]
          }
          event "Add FIFO": Value Change {
            n162 = event-data() -> ()  [unwired: 1 in, 6 out]
            n163 = case shown="True" "Add FIFO" {
              tunnel: w290 -> [_ w292]
              frame False {
              }
              frame True {
                n164 = Enqueue Element(queue=w292, element=cluster{"Enum":T2, variant} {"Enum"=enum."AddFIFO", variant}) -> ()  [unwired: 2 in, 3 out]
              }
            }
          }
          event "ClearFIFO": Value Change {
            n165 = event-data() -> ()  [unwired: 1 in, 6 out]
            n166 = case shown="True" "ClearFIFO" {
              tunnel: w294 -> [_ w296]
              frame False {
              }
              frame True {
                n167 = Enqueue Element(queue=w296, element=cluster{"Enum":T2, variant} {"Enum"=enum."ClrFIFO", variant}) -> ()  [unwired: 2 in, 3 out]
              }
            }
          }
          event "Save": Value Change {
            n168 = event-data() -> ()  [unwired: 1 in, 6 out]
            n169 = case shown="True" "Save" {
              tunnel: w299 -> [_ w301]
              frame False {
              }
              frame True {
                n170 = Enqueue Element(queue=w301, element=cluster{"Enum":T2, variant} {"Enum"=enum."Save", variant}) -> ()  [unwired: 2 in, 3 out]
              }
            }
          }
          event "Acquiring": Value Change {
            n171 = event-data() -> ()  [unwired: 1 in, 6 out]
          }
        }
      }
      n172 = while {
        tunnel: w24 -> [w68]
        tunnel: w25 -> [w65]
        stop <- w66 stop-if-true
        # "Data Process"
        n173 = call "GetFPGAStatus.vi"("FPGA in"=w65) -> ("FPGA out"=w64:refnum<queue>, "Demodulation"=w63:bool)  [unwired: 9 in, 4 out]
        n174 = case shown="True" w63 {
          tunnel: w68 -> [w70 w76]
          tunnel: w64 -> [w69 w75]
          frame False {
            n175 = call "DataProcessorRAW.vi"("FPGA in"=w69, "Queue in"=w70) -> ()  [unwired: 7 in]
          }
          frame True {
            n176 = local read "Averaging prefered"() -> (w73:bool)
            n177 = Select(t=w73, s="Auto MA selection", f="Averaging") -> (s? t:f=w71:bool)
            "Averaging" <- w71
            n178 = case shown="False" w71 {
              tunnel: w76 -> [w80 w82]
              tunnel: w75 -> [w79 w81]
              frame False {
                n179 = call "DataProcessorDEMBUT.vi"("Settling"="Settling at step time", "Filter Order"="Lockin filter order", "FPGA in"=w79, "DATA in"=w80) -> ()  [unwired: 8 in]
              }
              frame True {
                n180 = call "DataProcessorDEM.vi"("DATA in"=w82, "FPGA in"=w81) -> ()  [unwired: 6 in]
              }
            }
          }
        }
        n181 = Wait (ms)(milliseconds to wait=u32 50) -> ()  [unwired: 1 out]
        n182 = local read "exit"() -> (w66:bool)
      }
      n183 = while {
        tunnel: w25 -> [w37]
        tunnel: [w33] -> w27
        shift-right: [w32] -> w26
        shift-left: w24 -> [w38]
        stop <- w31 stop-if-true
        n184 = call "GetFPGAConnections.vi"("FPGA in"=w37) -> ("connection cluster"=w36:T4)  [unwired: 9 in, 1 out]
        n185 = local read "exit"() -> (w31:bool)
        n186 = Unbundle By Name(w36) -> ("DFAST ID"=w35:refnum<k16>, "DFAST error out"=w34:errorcluster)
        n187 = Wait (ms)(milliseconds to wait=u32 200) -> ()  [unwired: 1 out]
        n188 = while {
          tunnel: w35 -> [w52]
          tunnel: w38 -> [w49]
          shift-right: [w47] -> w33
          shift-left: w34 -> [w51]
          tunnel: [w46] -> w32
          shift-right: [w39] -> _
          shift-left: _ -> [w41]
          stop <- w42 stop-if-true
          # "UDP 2048 Data Fetch"
          n189 = UDP Read(connection ID=w52, max size (548)=3999 ("timeout ms (25000)"), timeout ms (25000)=200, 8:w51) -> (data out=w50:string, error out=w45:errorcluster)  [unwired: 3 out]
          n190 = Unbundle By Name(w45) -> ("status"=w44:bool)
          n191 = local read "exit"() -> (w43:bool)
          n192 = case shown="No Error" w45 {
            tunnel: w49 -> [w60 w62]
            tunnel: w50 -> [w58 _]
            tunnel: [w59 w62] -> w46
            tunnel: w41 -> [w57 _]
            tunnel: [w56 u32 0] -> w39
            frame No Error {
              n193 = Lossy Enqueue Element(queue=w60, element=w58) -> (queue out=w59:refnum<queue>)  [unwired: 1 in, 3 out]
              n194 = Add(x=u32 1, y=w57) -> (x+y=w56:u32)
            }
            frame Error {
            }
          }
          n195 = call <vilib>:"Clear Errors.vi"("error in (no error)"=w45, "specific error code to clear (0: all)"=56) -> ("error out"=w47:errorcluster)  [unwired: 4 in, 1 out]
          n196 = Not Equal To 0?(x=w39) -> (x != 0?=w40:bool)
          n197 = case shown="True" w40 {
            tunnel: w39 -> [_ _]
            frame False {
            }
            frame True {
            }
          }
          n198 = Compound Arithmetic op=OR(w44, w43) -> (w42:bool)
        }
      }
      n199 = call <vilib>:"Clear Errors.vi"("error in (no error)"=w27) -> ()  [unwired: 5 in, 2 out]
      n200 = Release Queue(queue=w26) -> ()  [unwired: 2 in, 3 out]
    }
  }
  n201 = flat-sequence {
    tunnel: w2 -> [w303]
    tunnel: [w303] -> w1
    tunnel: w1 -> [w304]
    frame #0 {
      n202 = Wait (ms)(milliseconds to wait=u32 500) -> ()  [unwired: 1 out]
    }
    frame #1 {
      n203 = call "DestroySEQ.vi"("FPGA out"=w304) -> ()  [unwired: 11 in]
    }
  }
  n204 = flat-sequence {
    tunnel: w3 -> [_]
    frame #0 {
      n205 = local write "exit"(FALSE) -> ()
    }
  }
